vi "robotArriveInAPosition.vi"(4 "AttackerAngle\nToTurnInDegrees":dbl, 6 "DistanceToConsiderRobotArrive":dbl, 7 "Target(x, y, orientation)":dbl[](array[numeric]), 8 "error in (no error)":errorcluster, 10 "Robot":refnum<class "Robot.lvclass">, 11 "Utilities in":refnum<class "Utilities.lvclass">) -> (0 "error out":errorcluster, 2 "arrive?":bool, 3 "Utilities out":refnum<class "Utilities.lvclass">)   [LabVIEW 2020, in "Utilities.lvclass"]
uses:
  Utilities.lvclass
  Robot_class/Robot.lvclass
  C:/RoboIME/SSL_AI/Object_class/Object.lvclass
  Robot_class/Robot.lvclass/Robot.ctl
  Object_class/Object.lvclass/Object.ctl
  <vilib>/Analysis/_algsub.llb/Real Vector Norm.vi
  <vilib>/Analysis/coordinate.llb/Wrap Angle (scalar).vi
  Robot_class/Read orientation.vi
  Object_class/Read position(x,y).vi
  <vilib>/Analysis/NI_AAL_Angle.lvlib
  <vilib>/Analysis/NI_AALPro.lvlib
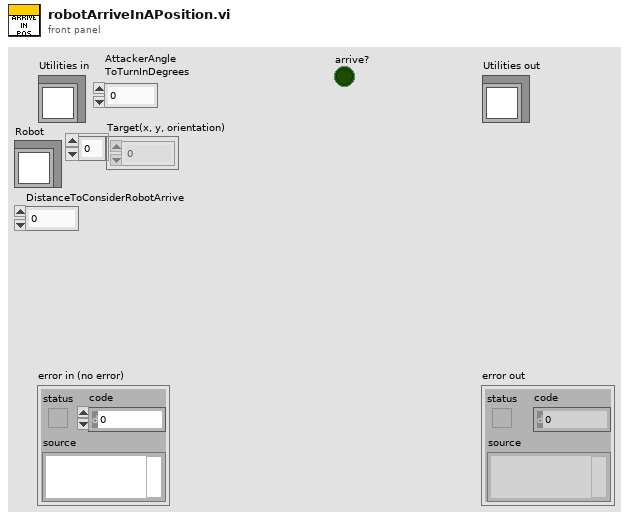
[diagram p1: front panel]
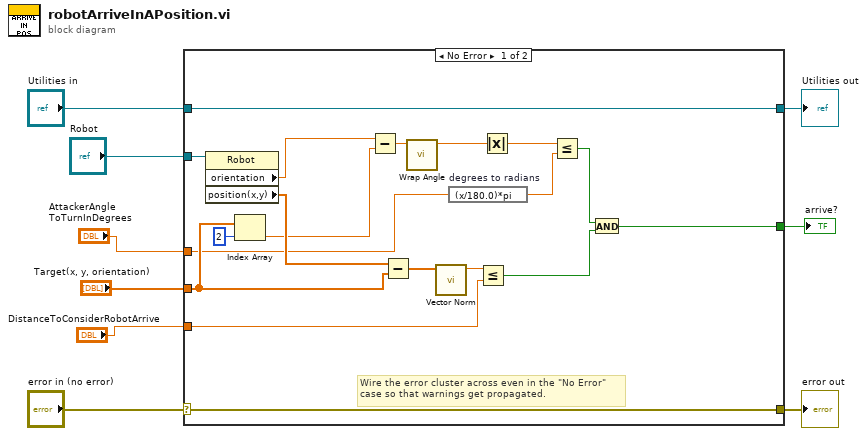
[diagram p0: block diagram]
diagram:
  n1 = case shown="No Error" "error in (no error)" {
    selector: "error in (no error)" -> [w27 w30]
    tunnel: [w27 w30] -> w8
    tunnel: [w28 w29] -> w6
    tunnel: "Utilities in" -> [w28 w29]
    tunnel: "Robot" -> [w17 _]
    tunnel: [w18 _] -> w4
    tunnel: "Target(x, y, orientation)" -> [w14 _]
    tunnel: "DistanceToConsiderRobotArrive" -> [w11 _]
    tunnel: "AttackerAngle\nToTurnInDegrees" -> [w10 _]
    frame No Error {
      # "Wire the error cluster across even in the \"No Error\"\ncase so that warnings get propagated."
      n2 = property class="Robot"(reference=w17) -> ("orientation"=w16:dbl, "position(x,y)"=w15:dbl[])  [unwired: 1 in, 2 out]
      n3 = Index Array(array=w14, index=2) -> (element=w12:dbl)
      n4 = Subtract(x=w16, y=w12) -> (x-y=w26:dbl)
      n5 = Subtract(x=w15, y=w14) -> (x-y=w22:dbl[])
      n6 = call-poly <vilib>:"Wrap Angle.vi"("angle in"=w26) -> ("angle out"=w25:dbl)  [unwired: 9 in, 1 out]
      n7 = call-poly <vilib>:"Vector Norm.vi"("Input Vector"=w22) -> ("norm"=w21:dbl)  [unwired: 9 in, 1 out]
      n8 = expression code="(x/180.0)*pi" "degrees to radians"(w10) -> (w23:dbl)
      n9 = Less Or Equal?(x=w21, y=w11) -> (x <= y?=w19:bool)
      n10 = Absolute Value(x=w25) -> (abs(x)=w24:dbl)
      n11 = Less Or Equal?(x=w24, y=w23) -> (x <= y?=w20:bool)
      n12 = And(x=w20, y=w19) -> (x .and. y?=w18:bool)
    }
    frame Error {
    }
  }
  "error out" <- w8
  "Utilities out" <- w6
  "arrive?" <- w4
